vi "Spartan HTTP VIT Close.vi"(8 "error in":errorcluster, 9 "Content":string, 10 "Header":string, 11 "HTTP session":T1 {"object data"."time" format="%0.2f"}) -> (0 "error out":errorcluster)   [LabVIEW 2011]
uses:
  Spartan HTTP Session.ctl
  ITK EXT/http/http_obj.llb/HTTP Session Data.ctl
  ITK EXT/utils/keyedarr.llb/Keyed Array.ctl
  Spartan HTTP Server Globals.vi
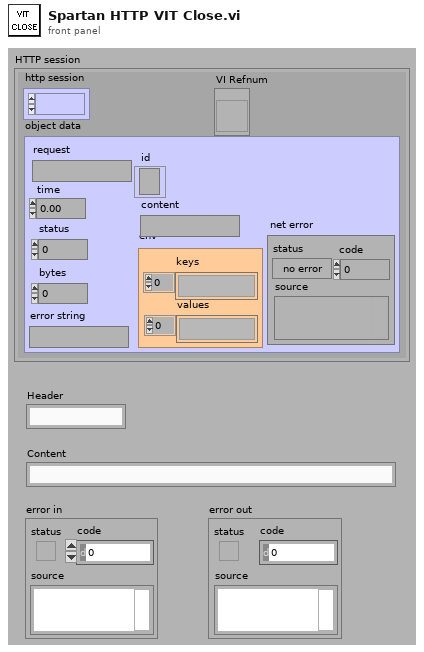
[diagram p1: front panel]
types:
  T1 = typedef "Spartan HTTP Session.ctl" = cluster{"http session":refnum<k1>, "object data":T2, "VI Refnum":refnum<vi>}
  T2 = typedef "HTTP Session Data.ctl" = cluster{"request":string, "time":dbl, "status":i32, "error string":string, "bytes":i32, "env":T3, "content":string, "id":refnum<k5>, "net error":errorcluster}
  T3 = typedef "Keyed Array.ctl" = cluster{"keys":string[], "values":string[]}
  T4 = typedef "Semaphore RefNum" = refnum<k1>
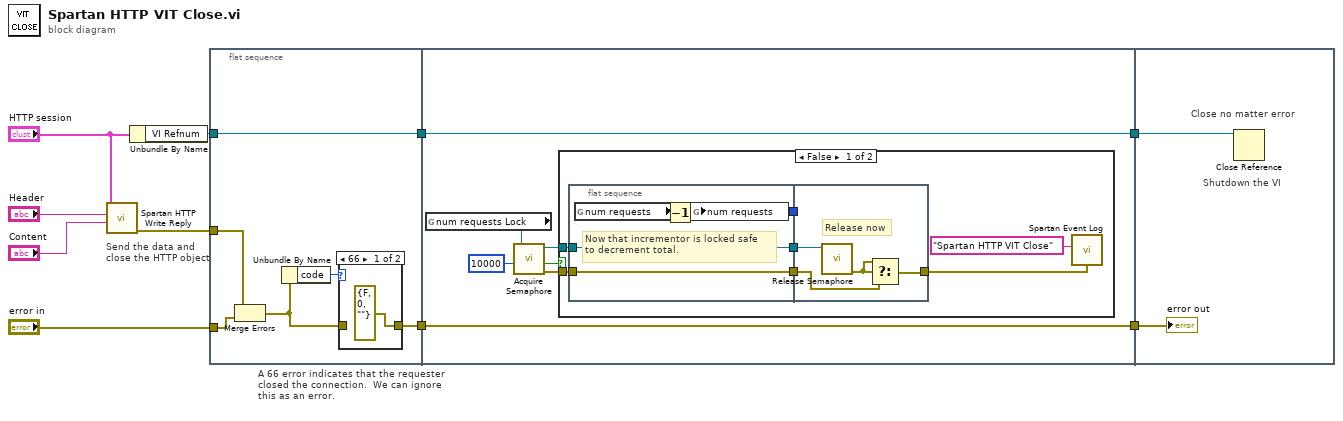
[diagram p0: block diagram]
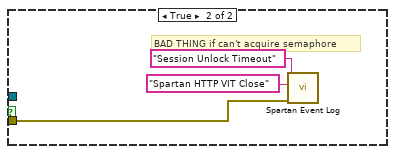
[diagram p3: hidden frame]
diagram:
  # "A 66 error indicates that the requester\nclosed the connection.  We can ignore\nthis as an error."
  # "Send the data and \nclose the HTTP object"
  n1 = call "Spartan HTTP Write Reply.vi"("content"="Content", "header"="Header", "http session"="HTTP session") -> ("error out"=w8:errorcluster)  [unwired: 1 in, 7 out]
  n2 = Unbundle By Name("HTTP session") -> ("VI Refnum"=w10:refnum<vi>)
  n3 = flat-sequence {
    tunnel: "error in" -> [w14]
    tunnel: w10 -> [w16]
    tunnel: [w16] -> w7
    tunnel: w8 -> [w15]
    tunnel: [w13] -> w5
    tunnel: w7 -> [w25]
    tunnel: [w25] -> w6
    tunnel: w5 -> [w19]
    tunnel: [w19] -> w4
    tunnel: w6 -> [w45]
    tunnel: w4 -> [w44]
    frame #0 {
      n4 = Merge Errors(w15, w14) -> (w11:errorcluster)
      n5 = Unbundle By Name(w11) -> ("code"=w12:i32)
      n6 = case shown="66" w12 {
        tunnel: [errorcluster {"status"=FALSE, "code"=0, "source"=""} ("error out") w18] -> w13
        tunnel: w11 -> [_ w18]
        frame 66 {
        }
        frame Default {
        }
      }
    }
    frame #1 {
      n7 = global read "Spartan HTTP Server Globals.vi" "num requests Lock"() -> (w24:T4)
      n8 = call <vilib>:"Acquire Semaphore.vi"("ms timeout (-1)"=10000, "semaphore"=w24) -> ("error out"=w21:errorcluster, "timed out"=w22:bool, "semaphore out"=w20:T4)  [unwired: 1 in, 2 out]
      n9 = case shown="False" w22 {
        tunnel: w21 -> [w30 w42]
        tunnel: w20 -> [w28 _]
        frame False {
          n10 = flat-sequence {
            tunnel: [w35] -> w32
            tunnel: [w34] -> w31
            tunnel: w30 -> [w34]
            tunnel: [w33] -> w29
            tunnel: w28 -> [w33]
            tunnel: w32 -> [_]
            tunnel: w31 -> [w38]
            tunnel: w29 -> [w40]
            tunnel: [w37] -> w27
            frame #0 {
              # "Now that incrementor is locked safe\nto decrement total."
              n11 = global read "Spartan HTTP Server Globals.vi" "num requests"() -> (w36:u32)
              n12 = Decrement(x=w36) -> (x-1=w35:u32)
              n13 = global write "Spartan HTTP Server Globals.vi" "num requests"(w35) -> ()
            }
            frame #1 {
              # "Release now"
              n14 = call <vilib>:"Release Semaphore.vi"("semaphore"=w40) -> ("error out"=w39:errorcluster)  [unwired: 1 in, 5 out]
              n15 = Select(t=w39, s=w39, f=w38) -> (s? t:f=w37:errorcluster)
            }
          }
          n16 = call "Spartan Event Log.vi"("error in (no error)"=w27, "module (\"\")"="Spartan HTTP VIT Close" ("name (unnamed)")) -> ()  [unwired: 3 in, 4 out]
        }
        frame True {
          # "BAD THING if can't acquire semaphore"
          n17 = call "Spartan Event Log.vi"("error in (no error)"=w42, "module (\"\")"="Spartan HTTP VIT Close" ("name (unnamed)"), "message (\"\")"="Session Unlock Timeout" ("name (unnamed)")) -> ()  [unwired: 2 in, 4 out]
        }
      }
    }
    frame #2 {
      # "Close no matter error"
      # "Shutdown the VI"
      n18 = Close Reference(reference=w45) -> ()  [unwired: 1 in, 1 out]
      "error out" <- w44
    }
  }
